vi "SensorsGetScheduledMessages.vi"(8 "error in (no error)":errorcluster, 11 "channel handle in":u64) -> (0 "error out":errorcluster, 1 "message handle out 4":u64, 2 "message handle out 3":u64, 3 "channel handle out":u64, 4 "message handle out 5":u64, 5 "message handle out 2":u64, 7 "message handle out 1":u64)   [LabVIEW 2023]
uses:
  <instrlib>/BTI429Lib/BTI429LV.lvlib
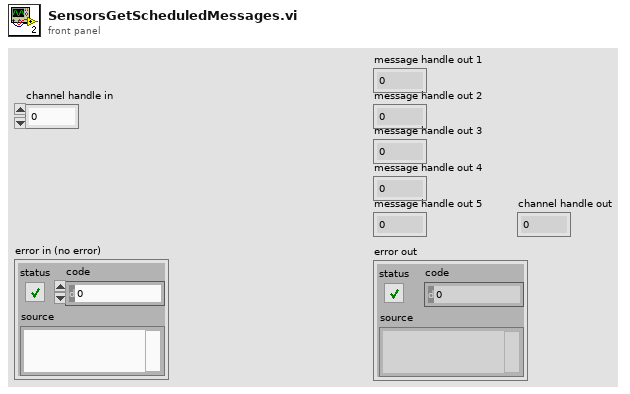
[diagram p1: front panel]
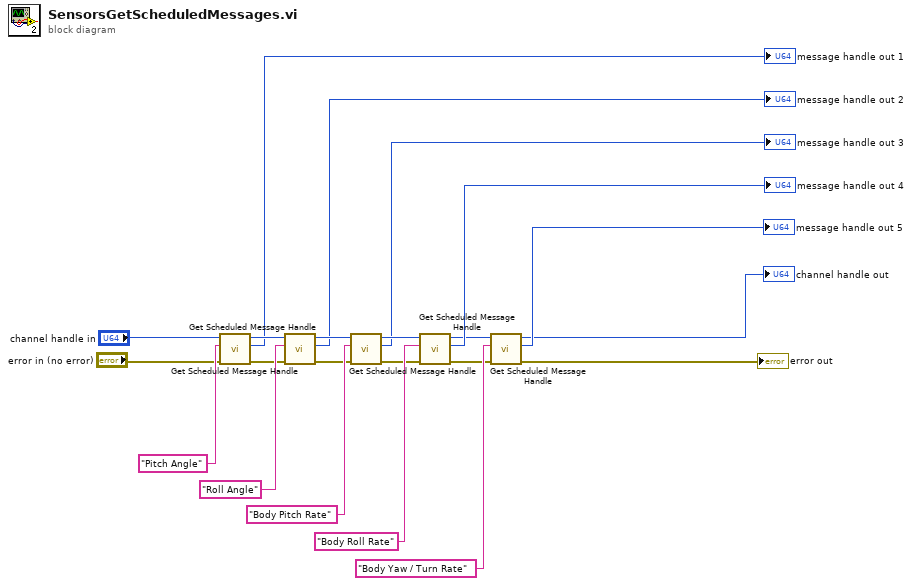
[diagram p0: block diagram]
diagram:
  n1 = call <instrlib>:"Get Scheduled Message Handle.vi"("error in (no error)"="error in (no error)", "message name"="Pitch Angle" ("msgname"), "channel handle in"="channel handle in") -> ("error out"=w8:errorcluster, "message handle out"=→"message handle out 1":u64, "channel handle out"=w7:u64)  [unwired: 6 in]
  n2 = call <instrlib>:"Get Scheduled Message Handle.vi"("error in (no error)"=w8, "message name"="Roll Angle" ("msgname"), "channel handle in"=w7) -> ("error out"=w10:errorcluster, "message handle out"=→"message handle out 2":u64, "channel handle out"=w11:u64)  [unwired: 6 in]
  n3 = call <instrlib>:"Get Scheduled Message Handle.vi"("error in (no error)"=w10, "message name"="Body Pitch Rate" ("msgname"), "channel handle in"=w11) -> ("error out"=w15:errorcluster, "message handle out"=→"message handle out 3":u64, "channel handle out"=w13:u64)  [unwired: 6 in]
  n4 = call <instrlib>:"Get Scheduled Message Handle.vi"("error in (no error)"=w15, "message name"="Body Roll Rate" ("msgname"), "channel handle in"=w13) -> ("error out"=w17:errorcluster, "message handle out"=→"message handle out 4":u64, "channel handle out"=w14:u64)  [unwired: 6 in]
  n5 = call <instrlib>:"Get Scheduled Message Handle.vi"("error in (no error)"=w17, "message name"="Body Yaw / Turn Rate" ("msgname"), "channel handle in"=w14) -> ("error out"=→"error out":errorcluster, "message handle out"=→"message handle out 5":u64, "channel handle out"=→"channel handle out":u64)  [unwired: 6 in]
